vi "Start Listener.vi"() -> ()   [LabVIEW 2010]
uses:
  Core SubVIs/Core SubVIs.lvlib
panel:
  in  "IP":string
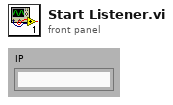
[diagram p1: front panel]
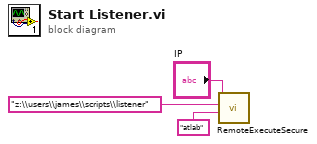
[diagram p0: block diagram]
diagram:
  n1 = call "RemoteExecuteSecure.vi"("User"="atlab", "Start Matlab Script"="z:\\users\\james\\scripts\\listener", "IP"="IP") -> ()  [unwired: 9 out]
